vi "Find All Children core.vi"(8 "error in (no error)":errorcluster, 9 "Panel":string, 11 "Panel Registry in":refnum<class "Panel Registry.lvclass">) -> (0 "error out":errorcluster, 2 "All Children":string[](array[string]))   [LabVIEW 2020, in "Panel.lvlib" / "Panel Registry.lvclass"]
uses:
  <vilib>/MGI/Panel Manager/Panel/Panel Registry/Panel Registry.lvclass
  <vilib>/MGI/Panel Manager/Panel/Panel Registry/Panel Registry.lvclass/Panel Registry.ctl
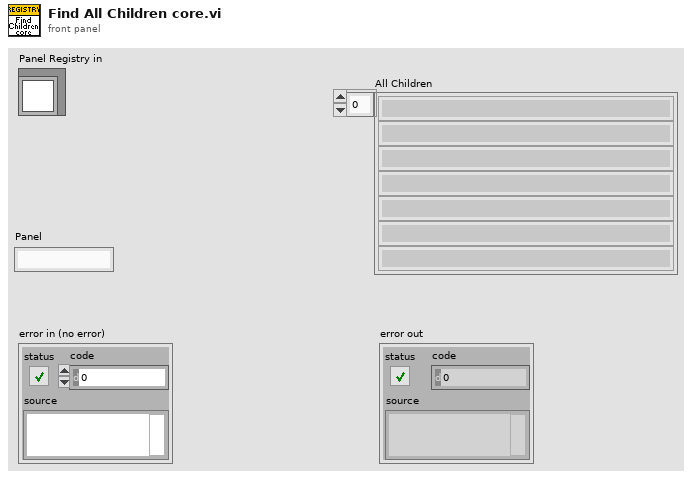
[diagram p1: front panel]
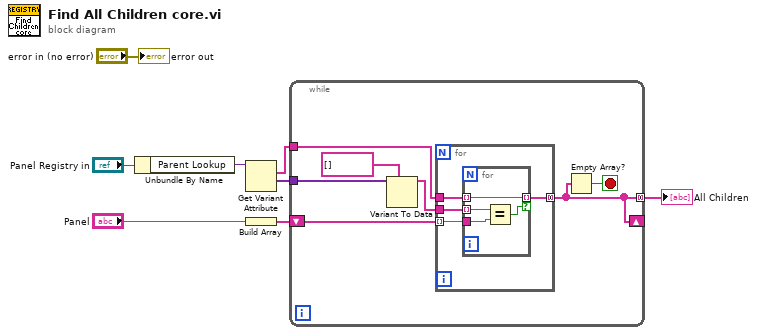
[diagram p0: block diagram]
diagram:
  n1 = Unbundle By Name("Panel Registry in") -> ("Parent Lookup"=w1:variant)
  n2 = Get Variant Attribute(Variant=w1) -> (names=w7:string[], values=w8:variant[])  [unwired: 3 in, 2 out]
  n3 = Build Array("Panel") -> (w5:string[])
  n4 = while {
    tunnel: w8 -> [w15]
    tunnel: w7 -> [w12]
    tunnel: [w9] -> w6 mode=concatenating
    shift-right: [w9] -> _
    shift-left: w5 -> [w10]
    stop <- w11 stop-if-true
    n5 = Variant To Data(type=string[] [] ("values"), Variant=w15) -> (data=w13:string[])  [unwired: 1 in, 1 out]
    n6 = for {
      tunnel: w13 -> [w17]
      tunnel: w10 -> [w16] mode=indexing
      tunnel: w12 -> [w19]
      tunnel: [w18] -> w9 mode=concatenating
      n7 = for {
        tunnel: w19 -> [w23] mode=indexing
        tunnel: [w23] -> w18 mode=indexing if=w20
        tunnel: w17 -> [w22] mode=indexing
        tunnel: w16 -> [w21]
        n8 = Equal?(x=w22, y=w21) -> (x = y?=w20:bool)
      }
    }
    n9 = Empty Array?(array=w9) -> (empty?=w11:bool)
  }
  "All Children" <- w6
  "error out" <- "error in (no error)"
